vi "ObjectCacher(VariantInterface).vi"(0 "key":string[](array[string]), 5 "array data source":variant[](array[variant]), 7 "typeKey(\"\" to use DataTypeDescription)":string, 11 "Enum(Get)":T1=enum."Get", 12 "type-postfix":string) -> (4 "values":variant[](array[variant]), 6 "names":string[](array[string]), 10 "found/Replace":bool[](array[boolean]), 14 "cacher":variant, 15 "error out":errorcluster)   [LabVIEW 2017]
uses:
  ObjectCacher-Operation.ctl
  <userlib>/_OpenG.lib/md5/md5.llb/MD5 Message Digest (Hexadecimal String)__ogtk.vi
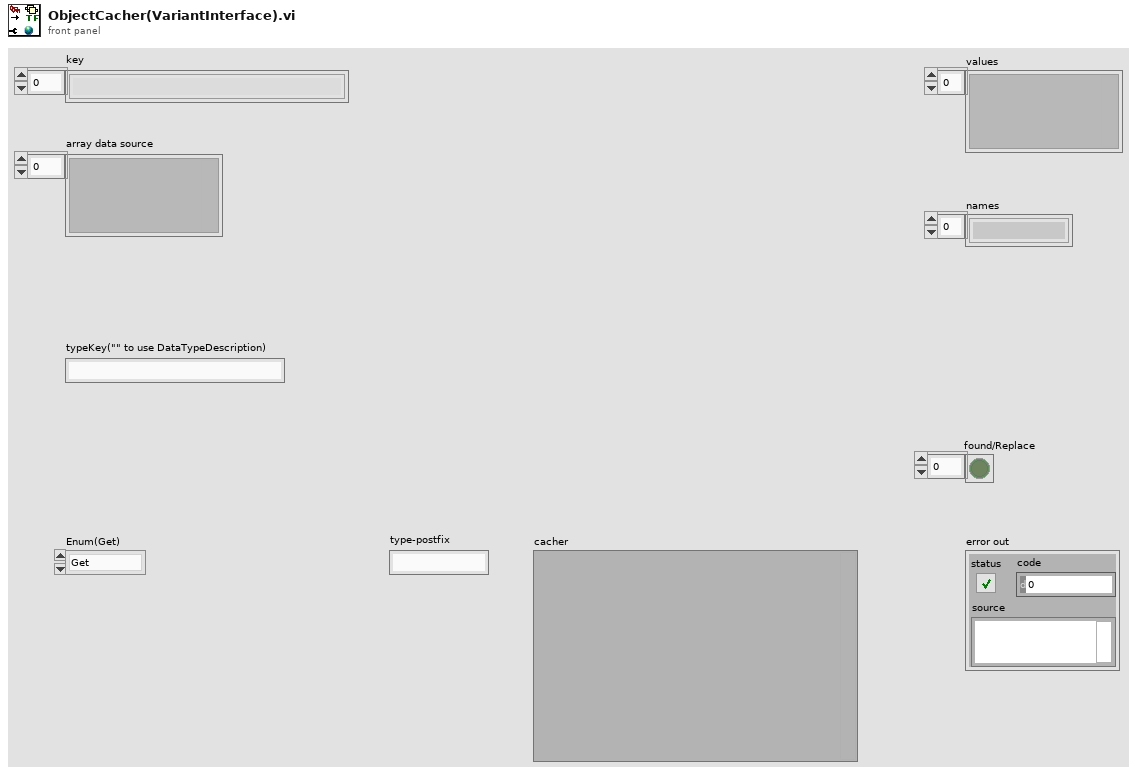
[diagram p1: front panel]
types:
  T1 = typedef "ObjectCacher-Operation.ctl" = enum16{"Reset", "Set", "Get", "Delete", "List", "<NONE>"}
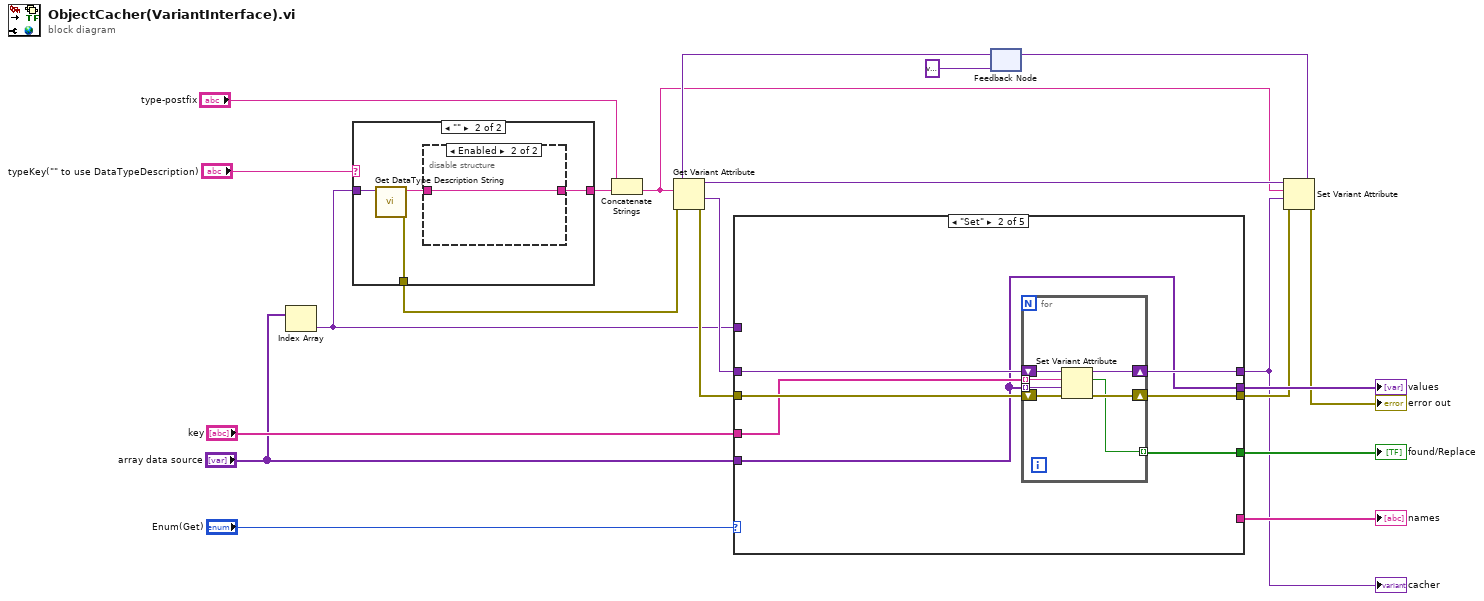
[diagram p0: block diagram]
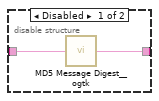
[diagram p3: hidden frame]
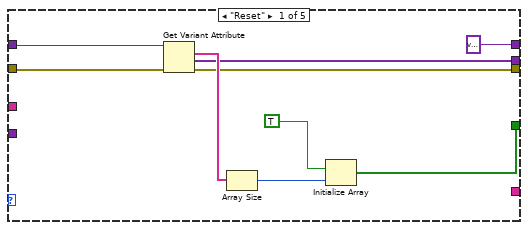
[diagram p4: hidden frame]
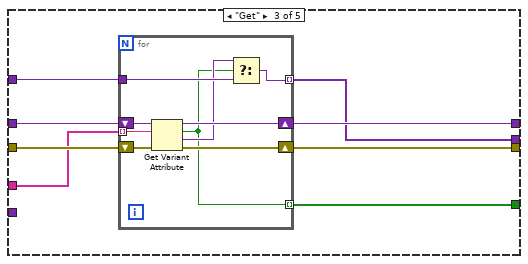
[diagram p5: hidden frame]
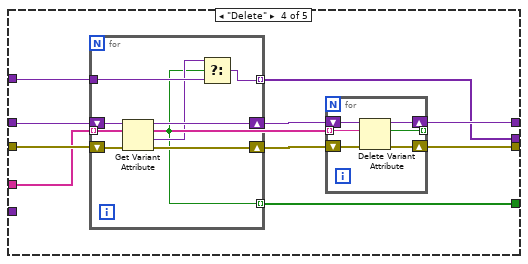
[diagram p6: hidden frame]
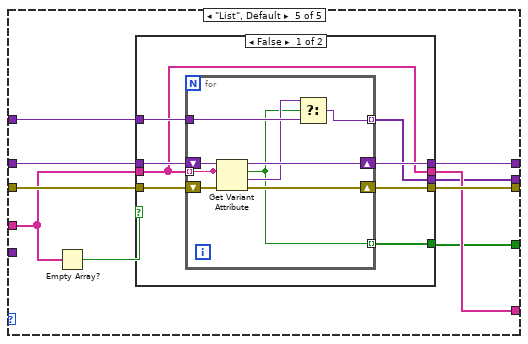
[diagram p7: hidden frame]
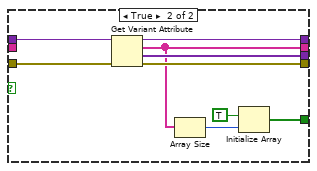
[diagram p8: hidden frame]
diagram:
  n1 = Index Array(array="array data source") -> (element=w2:variant)  [unwired: 1 in]
  n2 = case shown="\"\"" "typeKey(\"\" to use DataTypeDescription)" {
    selector: "typeKey(\"\" to use DataTypeDescription)" -> [w22 _]
    tunnel: [w22 w25] -> w15
    tunnel: w2 -> [_ w24]
    tunnel: [_ w23] -> w6
    frame Default {
    }
    frame "" {
      n3 = call "Get DataType Description String.vi"("Variant"=w24) -> ("error out"=w23:errorcluster, "String"=w26:string)  [unwired: 9 in]
      n4 = disable-structure shown="Enabled" {
        disable-tunnel: w26 -> [w28 w29]
        disable-tunnel: [w27 w29] -> w25
        frame Disabled {
          n5 = call-poly <userlib>:"MD5 Message Digest__ogtk.vi"("Message"=w28) -> ("MD5 Message Digest"=w27:string)
        }
        frame Enabled {
        }
      }
    }
  }
  n6 = Concatenate Strings("type-postfix", w15) -> (w8:string)
  n7 = feedback #1(variant) -> (w18:variant)
  n8 = Get Variant Attribute(Variant=w18, name=w8, error in=w6) -> (duplicate Variant=w11:variant, value=w16:variant, error out=w10:errorcluster)  [unwired: 1 in, 1 out]
  n9 = case shown="\"Set\"" "Enum(Get)" {
    tunnel: [w31 w39 w54 w70 w99] -> w20
    tunnel: [variant w45 w60 w78 w101] -> w1
    tunnel: w10 -> [w34 w44 w59 w76 w104]
    tunnel: [w32 w43 w58 w79 w103] -> w9
    tunnel: w16 -> [w33 w42 w57 w77 w102]
    tunnel: w2 -> [_ _ w55 w75 w96]
    tunnel: "key" -> [_ w40 w56 w74 w97]
    tunnel: [w30 w41 w53 w71 w95] -> w13
    tunnel: [_ _ _ _ w100] -> w12
    tunnel: "array data source" -> [_ w39 _ _ _]
    frame "Reset" {
      n10 = Get Variant Attribute(Variant=w33, error in=w34) -> (names=w37:string[], values=w31:variant[], error out=w32:errorcluster)  [unwired: 2 in, 1 out]
      n11 = Array Size(array=w37) -> (size(s)=w36:i32)
      n12 = Initialize Array(TRUE, w36) -> (w30:bool[])
    }
    frame "Set" {
      n13 = for {
        tunnel: w39 -> [w52] mode=indexing
        tunnel: w40 -> [w47] mode=indexing
        tunnel: [w46] -> w41 mode=indexing
        shift-right: [w49] -> w43
        shift-left: w44 -> [w50]
        shift-right: [w51] -> w45
        shift-left: w42 -> [w48]
        n14 = Set Variant Attribute(Variant=w48, name=w47, value=w52, error in=w50) -> (Variant out=w51:variant, replaced=w46:bool, error out=w49:errorcluster)
      }
    }
    frame "Get" {
      n15 = for {
        tunnel: w56 -> [w65] mode=indexing
        tunnel: [w61] -> w53 mode=indexing
        shift-right: [w67] -> w58
        shift-left: w59 -> [w68]
        shift-right: [w69] -> w60
        shift-left: w57 -> [w66]
        tunnel: w55 -> [w64]
        tunnel: [w62] -> w54 mode=indexing
        n16 = Get Variant Attribute(Variant=w66, name=w65, error in=w68) -> (duplicate Variant=w69:variant, found=w61:bool, value=w63:variant, error out=w67:errorcluster)  [unwired: 1 in]
        n17 = Select(t=w63, s=w61, f=w64) -> (s? t:f=w62:variant)
      }
    }
    frame "Delete" {
      n18 = for {
        tunnel: [w81] -> w71 mode=indexing
        shift-right: [w86] -> w72
        shift-left: w76 -> [w87]
        shift-right: [w88] -> w73
        shift-left: w77 -> [w85]
        tunnel: w75 -> [w84]
        tunnel: [w82] -> w70 mode=indexing
        tunnel: w74 -> [w80] mode=indexing
        n19 = Get Variant Attribute(Variant=w85, name=w80, error in=w87) -> (duplicate Variant=w88:variant, found=w81:bool, value=w83:variant, error out=w86:errorcluster)  [unwired: 1 in]
        n20 = Select(t=w83, s=w81, f=w84) -> (s? t:f=w82:variant)
      }
      n21 = for {
        tunnel: w74 -> [w91] mode=indexing
        tunnel: [w89] -> _ mode=indexing
        shift-right: [w93] -> w79
        shift-left: w72 -> [w94]
        shift-right: [w90] -> w78
        shift-left: w73 -> [w92]
        n22 = Delete Variant Attribute(4:w94, 6:w91, 7:w92) -> (0:w93:errorcluster, 2:w89:bool, 3:w90:variant)
      }
    }
    frame "List", Default {
      n23 = Empty Array?(array=w97) -> (empty?=w98:bool)
      n24 = case shown="False" w98 {
        tunnel: w104 -> [w111 w130]
        tunnel: [w109 w129] -> w103
        tunnel: w102 -> [w112 w128]
        tunnel: [w110 w127] -> w101
        tunnel: [w105 w124] -> w100
        tunnel: [w108 w126] -> w99
        tunnel: w97 -> [w105 _]
        tunnel: w96 -> [w107 _]
        tunnel: [w106 w125] -> w95
        frame False {
          n25 = for {
            tunnel: [w113] -> _ mode=indexing
            tunnel: [w114] -> w106 mode=indexing
            shift-right: [w119] -> w109
            shift-left: w111 -> [w120]
            shift-right: [w121] -> w110
            shift-left: w112 -> [w118]
            tunnel: w107 -> [w117]
            tunnel: [w115] -> w108 mode=indexing
            tunnel: w105 -> [w113] mode=indexing
            n26 = Get Variant Attribute(Variant=w118, name=w113, error in=w120) -> (duplicate Variant=w121:variant, found=w114:bool, value=w116:variant, error out=w119:errorcluster)  [unwired: 1 in]
            n27 = Select(t=w116, s=w114, f=w117) -> (s? t:f=w115:variant)
          }
        }
        frame True {
          n28 = Get Variant Attribute(Variant=w128, error in=w130) -> (duplicate Variant=w127:variant, names=w124:string[], values=w126:variant[], error out=w129:errorcluster)  [unwired: 2 in]
          n29 = Array Size(array=w124) -> (size(s)=w123:i32)
          n30 = Initialize Array(TRUE, w123) -> (w125:bool[])
        }
      }
    }
  }
  "values" <- w20
  "cacher" <- w1
  "found/Replace" <- w13
  "names" <- w12
  n31 = Set Variant Attribute(Variant=w11, name=w8, value=w1, error in=w9) -> (Variant out=w17:variant, error out=→"error out":errorcluster)  [unwired: 1 out]
  n32 = feedback-in #1(w17) -> ()
